vi "cs_loadStimParam.vi"(0 "error in (no error)":errorcluster) -> (5 "error out":errorcluster, 8 "Path":path, 14 "Total Trials":dbl, 15 "Trial Randomization":enum32{"50% exactly", "Radio Selection 2"}(radio), 16 "Go Trial S#":i32=3, 17 "NoGo Trial S#":i32=4, 18 "Stims 1":dbl[][](array[numeric]), 19 "Stims 2":dbl[][](array[numeric]))   [LabVIEW 2012]
uses:
  <vilib>/Utility/xml.llb/Read From XML File(array).vi
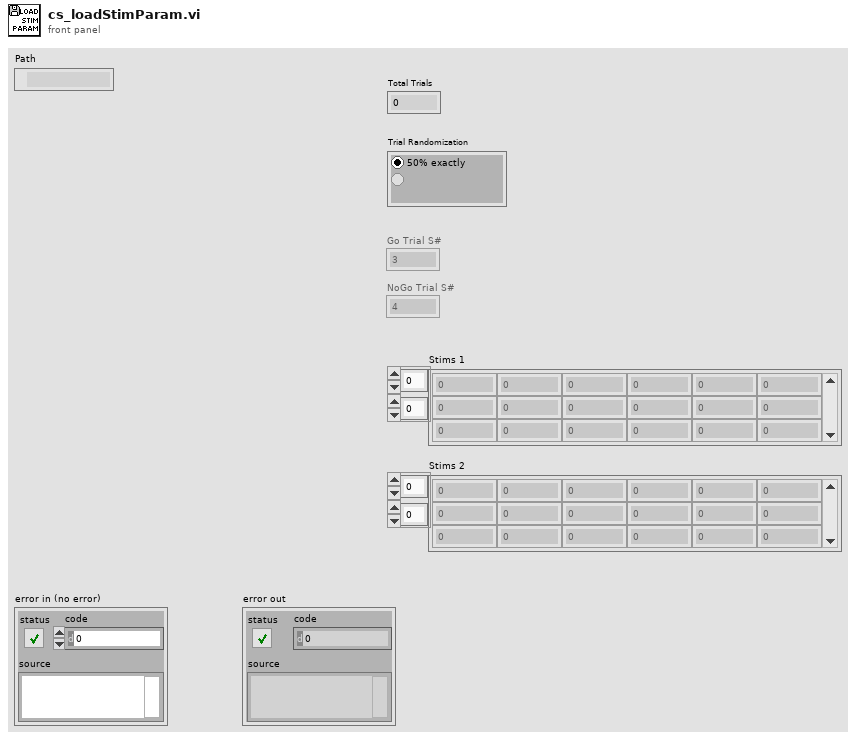
[diagram p1: front panel]
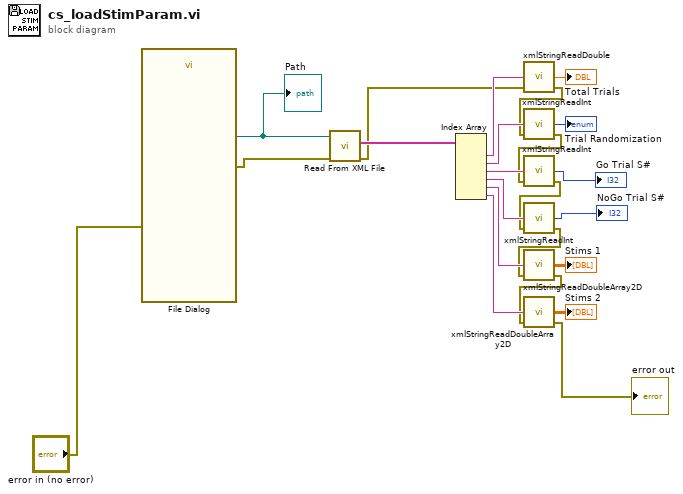
[diagram p0: block diagram]
diagram:
  n1 = call "File Dialog"("error in"="error in (no error)") -> ("selected path"=w22:path, "error out"=w21:errorcluster)  [unwired: 11 in, 2 out]
  "Path" <- w22
  n2 = call-poly <vilib>:"Read From XML File.vi"("error in (no error)"=w21, "XML File Path"=w22) -> ("error out"=w10:errorcluster, "XML Elements"=w23:string[])  [unwired: 7 in, 1 out]
  n3 = Index Array(array=w23) -> (element #1=w20:string, element #2=w18:string, element #3=w16:string, element #4=w15:string, element #5=w12:string, element #6=w11:string)  [unwired: 6 in]
  n4 = call "xmlStringReadDouble.vi"("error in (no error)"=w10, "String"=w20) -> ("error out"=w9:errorcluster, "Value"=→"Total Trials":dbl)  [unwired: 2 in]
  n5 = call "xmlStringReadInt.vi"("error in (no error)"=w9, "String"=w18) -> ("error out"=w8:errorcluster, "Value"=→"Trial Randomization":i32)  [unwired: 2 in]
  n6 = call "xmlStringReadInt.vi"("error in (no error)"=w8, "String"=w16) -> ("error out"=w7:errorcluster, "Value"=→"Go Trial S#":i32)  [unwired: 2 in]
  n7 = call "xmlStringReadInt.vi"("error in (no error)"=w7, "String"=w15) -> ("error out"=w6:errorcluster, "Value"=→"NoGo Trial S#":i32)  [unwired: 2 in]
  n8 = call "xmlStringReadDoubleArray2D.vi"("error in (no error)"=w6, "String"=w12) -> ("error out"=w5:errorcluster, "Value"=→"Stims 1":dbl[][])  [unwired: 2 in]
  n9 = call "xmlStringReadDoubleArray2D.vi"("error in (no error)"=w5, "String"=w11) -> ("error out"=→"error out":errorcluster, "Value"=→"Stims 2":dbl[][])  [unwired: 2 in]
